vi "TriggerTests_1.vi"() -> ()   [LabVIEW 2009]
uses:
  <vilib>/Utility/NIReport.llb/NI_report.lvclass
panel:
  in  "test2.5":bool
  out "Att Calibration":dbl[](array[numeric])
  in  "test 2.3b":bool
  in  "test 2.2":bool
  out "minims":dbl[](array[numeric])
  in  "test 2.1":bool
  in  "report file path":path=path "D:/CTA/IntegrationBoard/tmp/report.htm"
  in  "Instrument VISA in":T1={"AWG VISA"="81160A", "Oscilloscope  VISA "="DSO80204B", "Integration Board IP"="172.16.7.43", "connection ID"=refnum, "report out"=refnum}
  out "error out":errorcluster
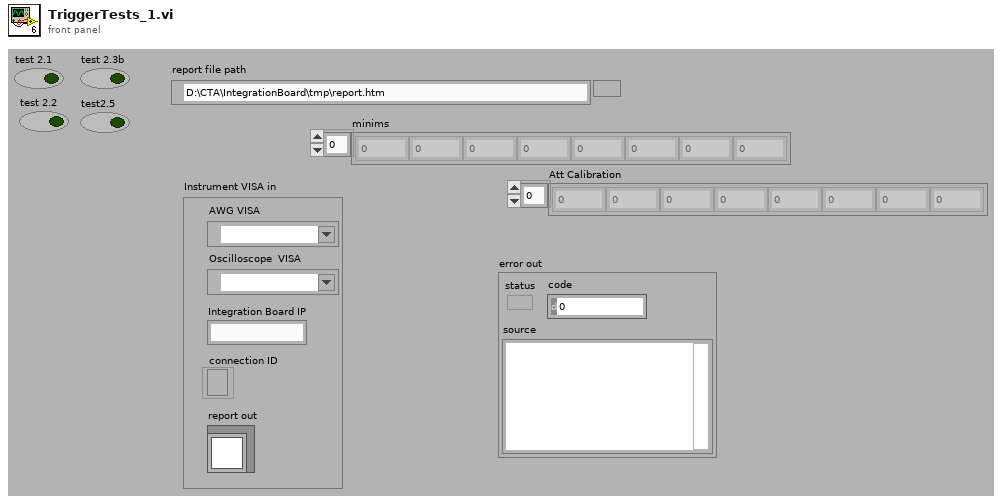
[diagram p1: front panel]
types:
  T1 = cluster{"AWG VISA":refnum<visa-resource-name>, "Oscilloscope  VISA ":refnum<visa-resource-name>, "Integration Board IP":string, "connection ID":refnum<k5>, "report out":refnum<class "NI_report.lvclass">}
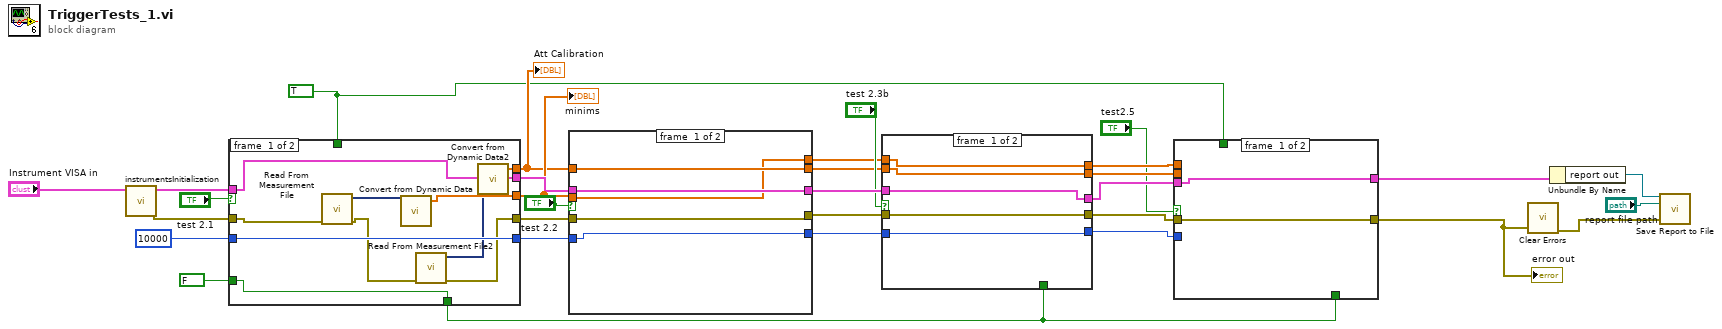
[diagram p0: block diagram]
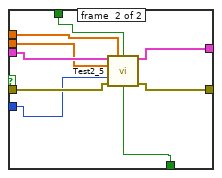
[diagram p2: hidden frame]
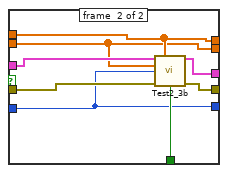
[diagram p3: hidden frame]
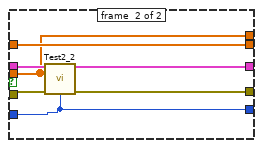
[diagram p4: hidden frame]
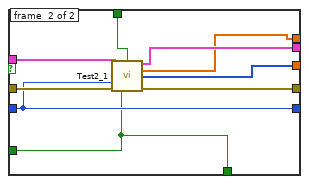
[diagram p5: hidden frame]
diagram:
  w1 = TRUE ("Report Enable")
  n1 = call "instrumentsInitialization.vi"("Instrument VISA in"="Instrument VISA in") -> ("error out"=w30:errorcluster, "Instrument VISA out"=w29:T1)  [unwired: 9 in]
  n2 = case shown="True" "test 2.1" {
    tunnel: w30 -> [w40 w50]
    tunnel: w29 -> [w41 w49]
    tunnel: 10000 ("Cycles Burst") -> [w37 w45]
    tunnel: [w35 w48] -> w26
    tunnel: [w41 w47] -> w24
    tunnel: [w38 w46] -> w23
    tunnel: [w37 w45] -> w21
    tunnel: [w33 w44] -> w13
    tunnel: [w32 w43] -> w5
    tunnel: FALSE ("L1 version") -> [w32 w43]
    tunnel: w1 -> [_ w42]
    frame #0 {
      n3 = call "Read From Measurement File"("error in (no error)"=w40) -> ("error out"=w36:errorcluster, "Signals"=w39:dynamicdata)  [unwired: 5 in, 4 out]
      n4 = call "Convert from Dynamic Data"("Dynamic Data Type"=w39) -> ("Array"=w38:dbl[])  [unwired: 3 in]
      n5 = call "Read From Measurement File2"("error in (no error)"=w36) -> ("error out"=w35:errorcluster, "Signals"=w34:dynamicdata)  [unwired: 5 in, 4 out]
      n6 = call "Convert from Dynamic Data2"("Dynamic Data Type"=w34) -> ("Array"=w33:dbl[])  [unwired: 3 in]
    }
    frame #1 {
      n7 = call "Test2_1.vi"("Instrument VISA in"=w49, "Report Enable"=w42, "Cycles Burst"=w45, "error in"=w50, "L1 version"=w43) -> ("Instrument VISA out"=w47:T1, "Calibration"=w44:dbl[], "L1 min values"=w46:i32[], "error out"=w48:errorcluster)  [unwired: 7 in]
    }
  }
  "minims" <- w23
  "Att Calibration" <- w13
  n8 = case shown="True" "test 2.2" {
    tunnel: w26 -> [w53 w62]
    tunnel: w24 -> [w55 w61]
    tunnel: [w55 w60] -> w18
    tunnel: w23 -> [w51 w56]
    tunnel: w21 -> [w54 w58]
    tunnel: [w53 w59] -> w17
    tunnel: [w54 w58] -> w15
    tunnel: [w52 w57] -> w14
    tunnel: w13 -> [w52 w57]
    tunnel: [w51 w56] -> w11
    frame #0 {
    }
    frame #1 {
      n9 = call "Test2_2.vi"("Instrument VISA in"=w61, "L1 min values"=w56, "error in"=w62, "Cycles Burst"=w58) -> ("Instrument VISA out"=w60:T1, "error out"=w59:errorcluster)  [unwired: 8 in, 2 out]
    }
  }
  n10 = case shown="True" "test 2.3b" {
    tunnel: w18 -> [w67 w75]
    tunnel: [w67 w74] -> w8
    tunnel: [w66 w73] -> w10
    tunnel: w17 -> [w66 w72]
    tunnel: w15 -> [w65 w70]
    tunnel: w14 -> [w64 w68]
    tunnel: w5 -> [_ w71]
    tunnel: w11 -> [w63 w69]
    tunnel: [w65 w70] -> w6
    tunnel: [w63 w69] -> w4
    tunnel: [w64 w68] -> w3
    frame #0 {
    }
    frame #1 {
      n11 = call "Test2_3b.vi"("Instrument VISA in"=w75, "Att minims"=w69, "Att Calibration ch"=w68, "Cycles Burst"=w70, "error in"=w72, "L1 version"=w71) -> ("Instrument VISA out"=w74:T1, "error out"=w73:errorcluster)  [unwired: 6 in, 2 out]
    }
  }
  n12 = case shown="True" "test2.5" {
    tunnel: w8 -> [w76 w83]
    tunnel: [w76 w84] -> w7
    tunnel: [w77 w85] -> w9
    tunnel: w10 -> [w77 w86]
    tunnel: w6 -> [_ w81]
    tunnel: w3 -> [_ w80]
    tunnel: w5 -> [_ w79]
    tunnel: w4 -> [_ w78]
    tunnel: w1 -> [_ w82]
    frame #0 {
    }
    frame #1 {
      n13 = call "Test2_5.vi"("Instrument VISA in"=w83, "Att minims"=w78, "Report Enable"=w82, "Att Calibration"=w80, "Cycles Burst"=w81, "error in"=w86, "L1 version"=w79) -> ("Instrument VISA out"=w84:T1, "error out"=w85:errorcluster)  [unwired: 5 in, 2 out]
    }
  }
  "error out" <- w9
  n14 = call <vilib>:"Clear Errors.vi"("error in (no error)"=w9) -> ("error out"=w20:errorcluster)  [unwired: 6 in]
  n15 = Unbundle By Name(w7) -> ("report out"=w28:refnum<class "NI_report.lvclass">)
  n16 = call-dynamic "Save Report to File.vi"("report in"=w28, "report file path"="report file path", "error in (no error)"=w20) -> ()  [unwired: 11 in, 2 out]
